vi "Read column.vi"(8 "error in (no error)":errorcluster, 11 "CellClick in":refnum<class "CellClick.lvclass">) -> (0 "error out":errorcluster, 2 "column":i32, 3 "CellClick out":refnum<class "CellClick.lvclass">)   [LabVIEW 2016, in "DataGrid.lvlib" / "CellClick.lvclass"]
uses:
  <userlib>/LabVIEWdotNetDataGrid/source/Events/CellClick/CellClick.lvclass
  <userlib>/LabVIEWdotNetDataGrid/source/Events/CellClick/CellClick.lvclass/CellClick.ctl
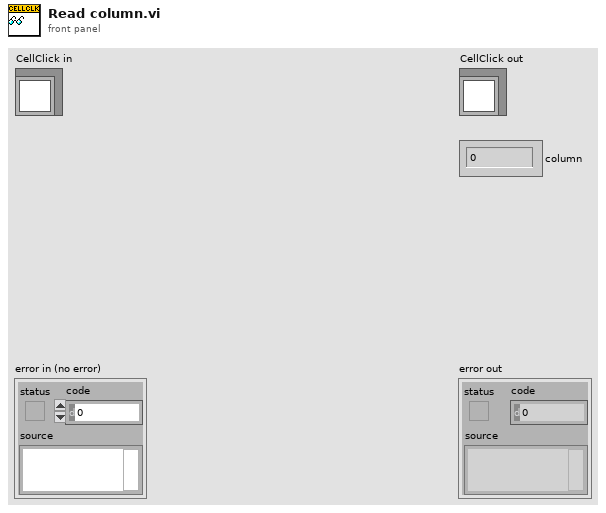
[diagram p1: front panel]
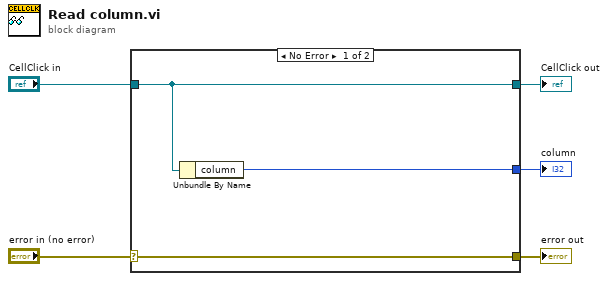
[diagram p0: block diagram]
diagram:
  n1 = case shown="No Error" "error in (no error)" {
    selector: "error in (no error)" -> [w8 w9]
    tunnel: [w8 w9] -> w4
    tunnel: [w7 w10] -> w2
    tunnel: "CellClick in" -> [w7 w10]
    tunnel: [w6 _] -> w1
    frame No Error {
      n2 = Unbundle By Name(w7) -> ("column"=w6:i32)
    }
    frame Error {
    }
  }
  "error out" <- w4
  "CellClick out" <- w2
  "column" <- w1
